vi "SetPoint.vi"(8 "error in (no error)":errorcluster, 10 "Point":refnum<class "Point.lvclass">, 11 "Picture in":refnum<class "Image.lvclass">) -> (0 "error out":errorcluster, 3 "Picture out":refnum<class "Image.lvclass">)   [LabVIEW 2021, in "Picture2D.lvlib" / "Image.lvclass"]
uses:
  Image.lvclass
  Picture2D/Picture2D.lvclass
  Point/Point.lvclass
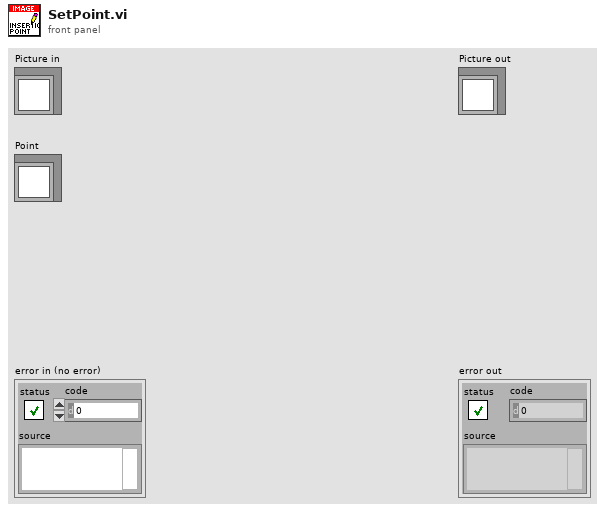
[diagram p1: front panel]
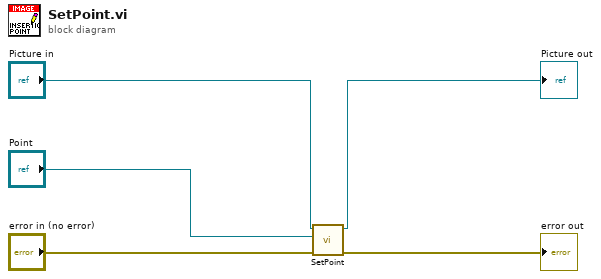
[diagram p0: block diagram]
diagram:
  n1 = call-parent "SetPoint.vi"("error in (no error)"="error in (no error)", "Point"="Point", "Picture2D in"="Picture in") -> ("error out"=→"error out":errorcluster, "Picture2D out"=→"Picture out":refnum<class "Image.lvclass">)  [unwired: 7 in]
